vi "FileHandler.vi"(8 "error in":errorcluster) -> (0 "error out":errorcluster)   [LabVIEW 2014]
uses:
  Controls/HeaderParameters.ctl
  Controls/DataPack.ctl
  Controls/ConfigFileWrite.ctl
  Controls/FGVisfileopen.ctl
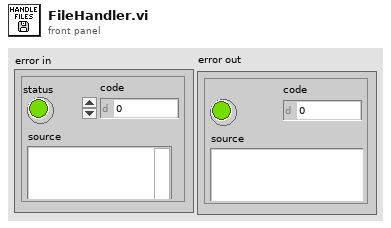
[diagram p1: front panel]
types:
  T1 = typedef "HeaderParameters.ctl" = cluster{"Property":string[], "Unit":string[], "Log Path":path}
  T2 = typedef "DataPack.ctl" = cluster{"DataPack Array":cluster{"Method":string, "PropertyName":string, "Value":string, "Display?":string, "Unit":string}[], "current time":timestamp}
  T3 = typedef "ConfigFileWrite.ctl" = cluster{"Headers":string[], "TableContent":string[][], "PathConfig":path}
  T4 = typedef "FGVisfileopen.ctl" = enum16{"Read", "Write"}
  T5 = typedef "FHandlerClusterTypedef.ctl" = cluster{"File Variant":variant, "FileHandler Enum":T6}
  T6 = typedef "FHandlerEnumTypedef.ctl" = enum16{"InitLog", "CommentLog", "WriteExperimental", "WriteRGA", "WriteAccelerator", "WriteInstrument", "ClearLog", "ReadConfig", "WriteConfig", "ExitFH"}
  T7 = cluster{"Method":string, "PropertyName":string, "Value":string, "Display?":string, "Unit":string}[]
  T8 = cluster{"Method":string, "PropertyName":string, "Value":string, "Display?":string, "Unit":string}
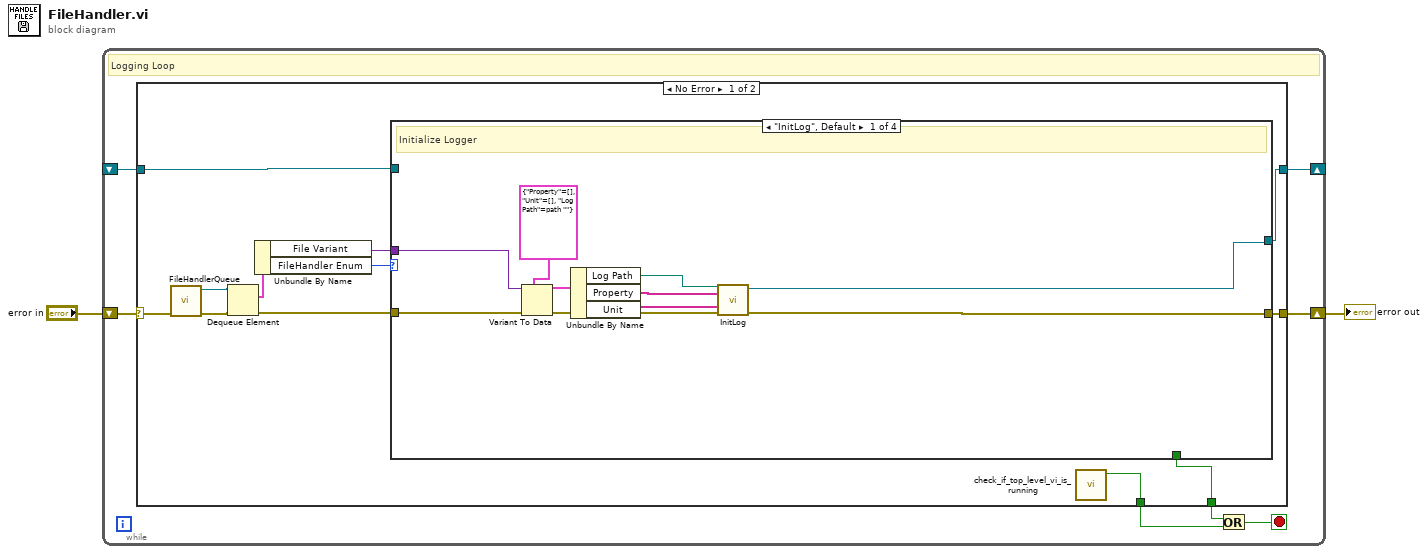
[diagram p0: block diagram]
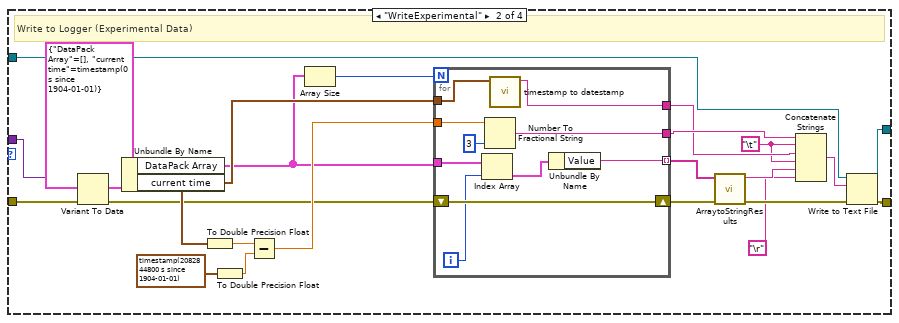
[diagram p2: hidden frame]
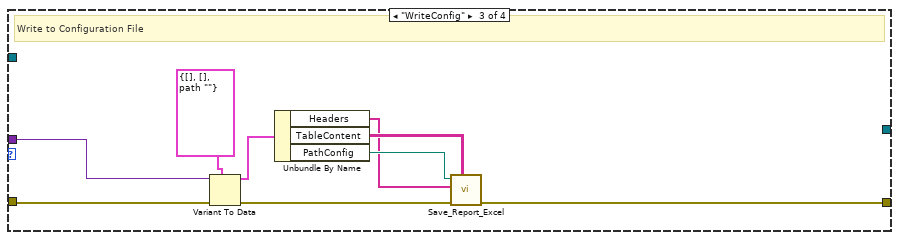
[diagram p3: hidden frame]
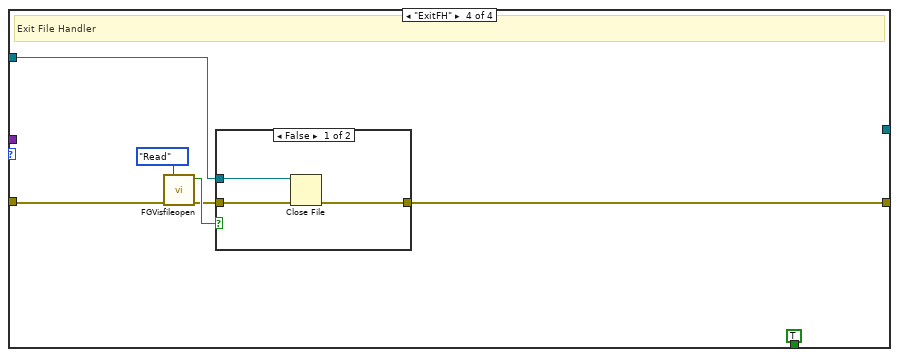
[diagram p4: hidden frame]
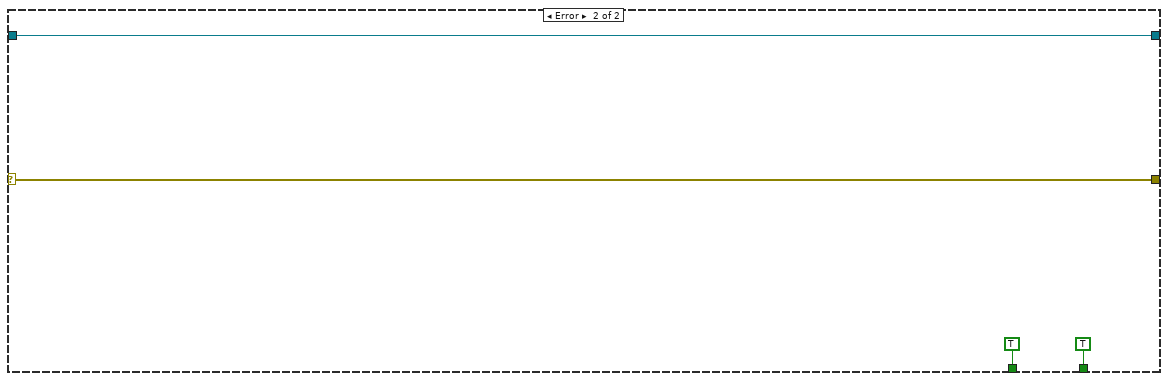
[diagram p6: hidden frame]
diagram:
  n1 = while {
    shift-right: [w9] -> w1
    shift-left: "error in" -> [w8]
    shift-right: [w7] -> _
    shift-left: _ -> [w6]
    stop <- w5 stop-if-true
    # "Logging Loop"
    n2 = case shown="No Error" w8 {
      selector: w8 -> [w11 w85]
      tunnel: [w15 w85] -> w9
      tunnel: [w10 TRUE] -> w4
      tunnel: [w14 w87] -> w7
      tunnel: w6 -> [w13 w87]
      tunnel: [w12 TRUE ("stop?")] -> w3
      frame No Error {
        n3 = call "FileHandlerQueue.vi"("error in"=w11) -> ("error out"=w21:errorcluster, "queue out"=w20:refnum<queue>)  [unwired: 8 in]
        n4 = Dequeue Element(queue=w20, error in (no error)=w21) -> (element=w19:T5, error out=w17:errorcluster)  [unwired: 1 in, 2 out]
        n5 = Unbundle By Name(w19) -> ("File Variant"=w16:variant, "FileHandler Enum"=w18:T6)
        n6 = case shown="\"InitLog\", Default" w18 {
          tunnel: [w31 w54 w69 w74] -> w15
          tunnel: w17 -> [w29 w52 w73 w75]
          tunnel: [_ _ _ TRUE] -> w10
          tunnel: w16 -> [w30 w32 w72 _]
          tunnel: [w27 w53 _ _] -> w14
          tunnel: w13 -> [_ w50 _ w79]
          frame "InitLog", Default {
            # "Initialize Logger"
            n7 = Variant To Data(error in=w29, type=T1 {"Property"=[], "Unit"=[], "Log Path"=path ""} ("Header Parameters"), Variant=w30) -> (data=w26:T1, error out=w28:errorcluster)
            n8 = Unbundle By Name(w26) -> ("Log Path"=w24:path, "Property"=w23:string[], "Unit"=w22:string[])
            n9 = call "InitLog.vi"("error control"=w28, "Unit"=w22, "Property"=w23, "file path (use dialog)"=w24) -> ("error indicator"=w31:errorcluster, "refnum out"=w27:refnum<file>)  [unwired: 6 in]
          }
          frame "WriteExperimental" {
            w39 = "\t"
            # "Write to Logger (Experimental Data)"
            n10 = Variant To Data(error in=w52, type=T2 {"DataPack Array"=[], "current time"=timestamp(0 s since 1904-01-01)}, Variant=w32) -> (data=w47:T2, error out=w33:errorcluster)
            n11 = Unbundle By Name(w47) -> ("DataPack Array"=w34:T7, "current time"=w42:timestamp)
            n12 = To Double Precision Float(number=w42) -> (double precision float=w46:dbl)
            n13 = To Double Precision Float(number=timestamp(2082844800 s since 1904-01-01)) -> (double precision float=w45:dbl)
            n14 = Subtract(x=w46, y=w45) -> (x-y=w43:dbl)
            n15 = Array Size(array=w34) -> (size(s)=w36:i32)
            n16 = for {
              N: w36 -> [_]
              shift-right: [w64] -> w49
              shift-left: w33 -> [w64]
              tunnel: w34 -> [w62]
              tunnel: [w59] -> w41
              tunnel: [w60] -> w48 mode=indexing
              tunnel: [w58] -> w40
              tunnel: w43 -> [w56]
              tunnel: w42 -> [w55]
              i -> [w63]
              n17 = Index Array(array=w62, index=w63) -> (element=w61:T8)
              n18 = Number To Fractional String(number=w56, precision (6)=i16 3) -> (F-format string=w59:string)  [unwired: 2 in]
              n19 = call "timestamp to datestamp.vi"("time stamp"=w55) -> ("remaining string"=w58:string)  [unwired: 9 in, 1 out]
              n20 = Unbundle By Name(w61) -> ("Value"=w60:string)
            }
            n21 = call "ArraytoStringResults.vi"("Array"=w48) -> ("String"=w38:string)  [unwired: 10 in]
            n22 = Concatenate Strings(w41, w39, w40, w39, w38, "\r") -> (w51:string)
            n23 = Write to Text File(file (use dialog)=w50, text=w51, error in=w49) -> (refnum out=w53:refnum<file>, error out=w54:errorcluster)  [unwired: 1 in, 1 out]
          }
          frame "WriteConfig" {
            # "Write to Configuration File"
            n24 = Variant To Data(error in=w73, type=T3 {"Headers"=[], "TableContent"=[], "PathConfig"=path ""}, Variant=w72) -> (data=w71:T3, error out=w70:errorcluster)
            n25 = Unbundle By Name(w71) -> ("Headers"=w66:string[], "TableContent"=w67:string[][], "PathConfig"=w68:path)
            n26 = call "Save_Report_Excel.vi"("Data In"=w67, "Error In"=w70, "Headers"=w66, "Report File Path In"=w68) -> ("Error Out"=w69:errorcluster)  [unwired: 6 in, 1 out]
          }
          frame "ExitFH" {
            # "Exit File Handler"
            n27 = call "FGVisfileopen.vi"("error in"=w75, "Read/Write?"=FGVisfileopen."Read" ("Write from FGV or Read from FGV?")) -> ("error out"=w76:errorcluster, "Output Value"=w77:bool)  [unwired: 8 in]
            n28 = case shown="False" w77 {
              tunnel: w76 -> [w83 w84]
              tunnel: [w82 w84] -> w74
              tunnel: w79 -> [w81 _]
              frame False {
                n29 = Close File(refnum=w81, error in=w83) -> (error out=w82:errorcluster)  [unwired: 1 out]
              }
              frame True {
              }
            }
          }
        }
        n30 = call "check_if_top_level_vi_is_running.vi"() -> ("stop?"=w12:bool)  [unwired: 10 in, 1 out]
      }
      frame Error {
      }
    }
    n31 = Or(x=w4, y=w3) -> (x .or. y?=w5:bool)
  }
  "error out" <- w1
